vi "SpecAn Preset.vi"(0 "VISA In":refnum<visa-resource-name>, 5 "Error In":errorcluster, 7 "Delay (ms)":u32=1500) -> (14 "VISA Out":refnum<visa-resource-name>, 19 "Error Out":errorcluster)   [LabVIEW 2015]
uses:
  Controls/FGV Action SpecAn Model.ctl
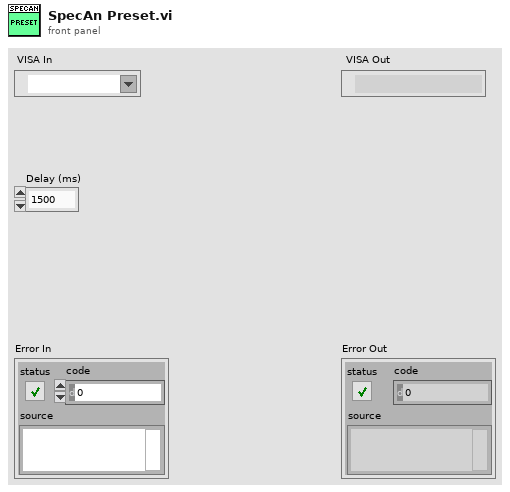
[diagram p1: front panel]
types:
  T1 = typedef "FGV Action SpecAn Model.ctl" = enum16{"Get", "Set"}
  T2 = typedef "SpecAn Model.ctl" = enum16{"E4440", "N9030"}
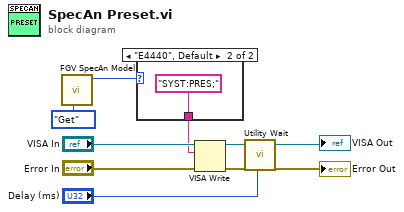
[diagram p0: block diagram]
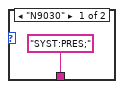
[diagram p2: hidden frame]
diagram:
  n1 = call "FGV SpecAn Model.vi"("Action"=FGV_Action_SpecAn_Model."Get") -> ("SA Model"=w1:T2)  [unwired: 6 in, 1 out]
  n2 = case shown="\"E4440\", Default" w1 {
    tunnel: ["SYST:PRES;" ("write buffer") "SYST:PRES;" ("write buffer")] -> w7
    frame "N9030" {
    }
    frame "E4440", Default {
    }
  }
  n3 = VISA Write(VISA resource name="VISA In", write buffer=w7, error in (no error)="Error In") -> (VISA resource name out=→"VISA Out":refnum<visa-resource-name>, error out=w6:errorcluster)  [unwired: 1 out]
  n4 = call "Utility Wait.vi"("Error In"=w6, "Wait (ms)"="Delay (ms)") -> ("Error Out"=→"Error Out":errorcluster)  [unwired: 17 in]
